vi "DriveForTime.vi"(7 "RobotDriveRef":T1, 8 "error in (no error)":errorcluster, 9 "SubSystem Data":T10, 10 "Control Mode":T8, 11 "Cluster":cluster{"Start Time (ms)":u32, "Iterations":i32}) -> (0 "error out":errorcluster, 1 "RobotDriveRef Out":T1, 2 "Wait":dbl, 3 "Finished":bool, 4 "Left Setpoint":dbl, 6 "Right Setpoint":dbl)   [LabVIEW 2015]
uses:
  Drive Setpoints.ctl
  Drive Operations.ctl
  Advanced Drive VIs/RobotDrive Type Def.ctl
  <vilib>/Rock Robotics/WPI/MotorControl/WPI_MotorControlDeviceRef.ctl
  <vilib>/Rock Robotics/WPI/MotorControl/WPI_MotorControlType.ctl
  <vilib>/Rock Robotics/SystemInterfaces/DIO/FPGA_DIOPWMChannel.ctl
  <vilib>/Rock Robotics/WPI/PWM/WPI_PWMDeadband.ctl
  <vilib>/Rock Robotics/WPI/CAN/Jaguar/SubVIs/WPI_CANJaguar_ControlMode.ctl
  <vilib>/Rock Robotics/WPI/CAN/TalonSRX/WPI_CANTalonSRX_APIControlMode.ctl
  Advanced Drive VIs/Drive Motor Settings.ctl
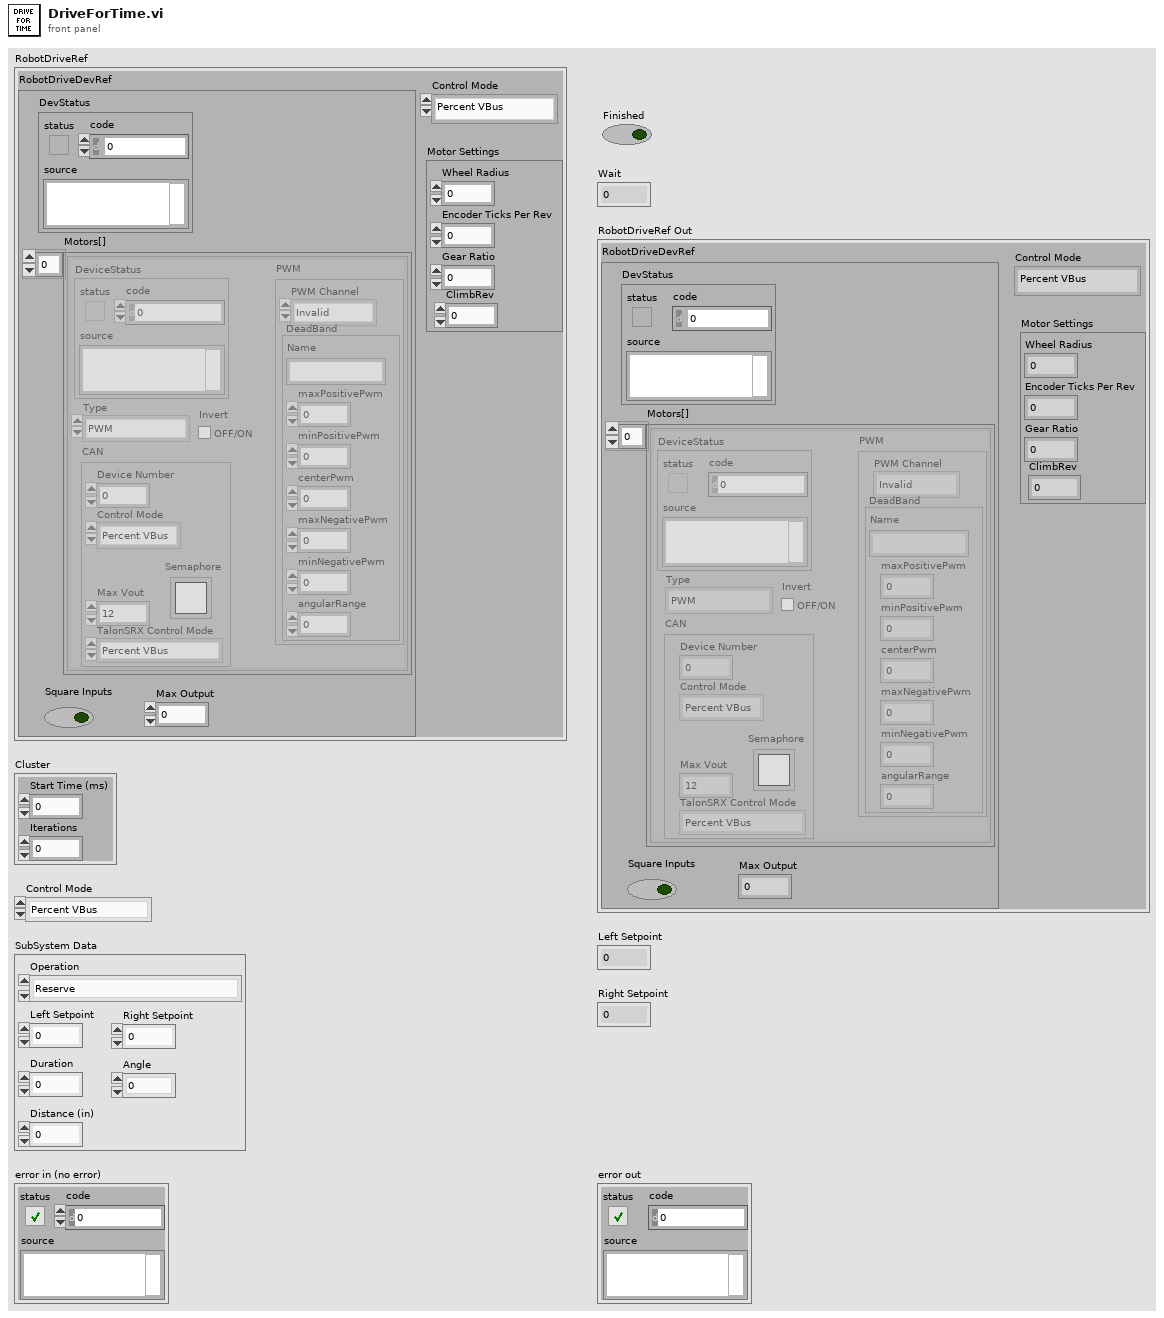
[diagram p1: front panel]
types:
  T1 = typedef "RobotDrive Type Def.ctl" = cluster{"RobotDriveDevRef":cluster{"DevStatus":errorcluster, "Motors[]":T2[], "Square Inputs":bool, "Max Output":dbl}, "Control Mode":T8, "Motor Settings":T9}
  T2 = typedef "WPI_MotorControlDeviceRef.ctl" = cluster{"DeviceStatus":errorcluster, "Type":T3, "PWM":cluster{"PWM Channel":T4, "DeadBand":T5}, "CAN":cluster{"Device Number":u8, "Control Mode":T6, "Semaphore":T7, "Max Vout":dbl, "TalonSRX Control Mode":T8}, "Invert":bool}
  T3 = typedef "WPI_MotorControlType.ctl" = enum16{"PWM", "CAN", "CANTalonSRX"}
  T4 = typedef "FPGA_DIOPWMChannel.ctl" = enum8{"PWM 0", "PWM 1", "PWM 2", "PWM 3", "PWM 4", "PWM 5", "PWM 6", "PWM 7", "PWM 8", "PWM 9", "PWM MXP 0", "PWM MXP 1", "PWM MXP 2", "PWM MXP 3", "PWM MXP 4", "PWM MXP 5", "PWM MXP 6", "PWM MXP 7", "PWM MXP 8", "PWM MXP 9", "Invalid"}
  T5 = typedef "WPI_PWMDeadband.ctl" = cluster{"Name":string, "maxPositivePwm":i32, "minPositivePwm":i32, "centerPwm":i32, "maxNegativePwm":i32, "minNegativePwm":i32, "angularRange":u16}
  T6 = typedef "WPI_CANJaguar_ControlMode.ctl" = enum8{"Percent VBus", "Current", "Speed", "Position", "Voltage"}
  T7 = typedef "Semaphore RefNum" = refnum<k1>
  T8 = typedef "WPI_CANTalonSRX_APIControlMode.ctl" = enum8{"Percent VBus", "Speed", "Position", "Slave", "Unchanged / Invalid", "Voltage Compensation", "Current", "Motion Profile"}
  T9 = typedef "Drive Motor Settings.ctl" = cluster{"Wheel Radius":dbl, "Encoder Ticks Per Rev":dbl, "Gear Ratio":dbl, "ClimbRev":dbl}
  T10 = typedef "Drive Setpoints.ctl" = cluster{"Operation":T11, "Left Setpoint":dbl, "Right Setpoint":dbl, "Duration":dbl, "Angle":dbl, "Distance (in)":dbl}
  T11 = typedef "Drive Operations.ctl" = enum16{"Reserve", "Read Current", "Immediate", "Drive for Time", "Drive for Distance", "Turn Degrees"}
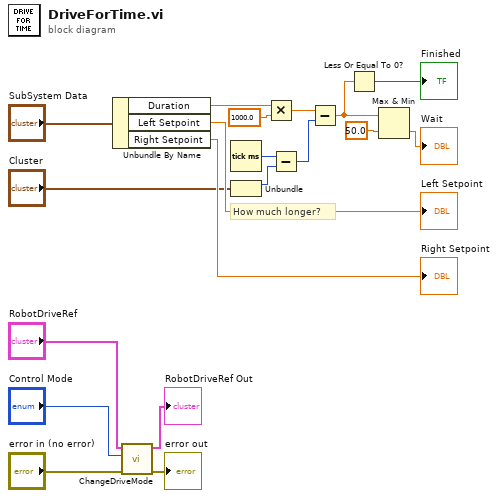
[diagram p0: block diagram]
diagram:
  # "How much longer?"
  n1 = Unbundle By Name("SubSystem Data") -> ("Duration"=w17:dbl, "Left Setpoint"=→"Left Setpoint":dbl, "Right Setpoint"=→"Right Setpoint":dbl)
  n2 = call "ChangeDriveMode.vi"("error in (no error)"="error in (no error)", "Control Mode"="Control Mode", "RobotDriveRef"="RobotDriveRef") -> ("error out"=→"error out":errorcluster, "RobotDriveRef Out"=→"RobotDriveRef Out":T1)  [unwired: 7 in]
  n3 = Tick Count (ms)() -> (millisecond timer value=w1:u32)
  n4 = Unbundle("Cluster") -> ("Start Time (ms)"=w6:u32)  [unwired: 1 out]
  n5 = Multiply(x=w17, y=1000.0) -> (x*y=w3:dbl)
  n6 = Subtract(x=w1, y=w6) -> (x-y=w2:u32)
  n7 = Subtract(x=w3, y=w2) -> (x-y=w8:dbl)
  n8 = Less Or Equal To 0?(x=w8) -> (x <= 0?=→"Finished":bool)
  n9 = Max & Min(x=w8, y=50.0) -> (min(x,y)=→"Wait":dbl)  [unwired: 1 out]
